vi "XIPIN_MicroBlaze_Debug_Module_(MDM)_3_2.vi"   [LabVIEW 2017]
doc: "Debug module for MicroBlaze Soft Processor.\n------------------------------------\n<b>Need License</b> : No\n<b>Interface</b> : AXI4 AXI4-Stream"
uses:
  <vilib>/rvi/XilinxIP/XIPIN_XNode/niFpgaXIPIN.xnode
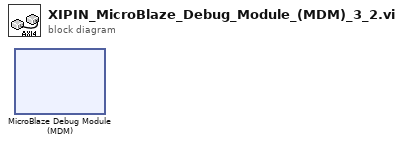
[diagram p0: block diagram]
diagram:
  n1 = xnode ("MicroBlaze Debug Module (MDM)")() -> ()
